vi "TROUBLESHOOTING.vi"() -> ()   [LabVIEW 2017]
uses:
  C:/Users/Admin/Desktop/Sensitive EQE Stuff/S-EQE (YJ)/Mono vi (YJ)/Cornerstone.dll
  Cornerstone.dll
panel:
  out "sendCommand":bool
  out "getResponse":string
  out "Mono Connected?":bool
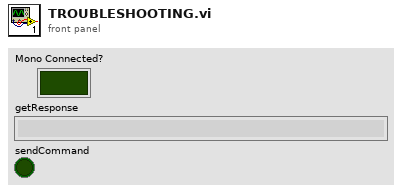
[diagram p1: front panel]
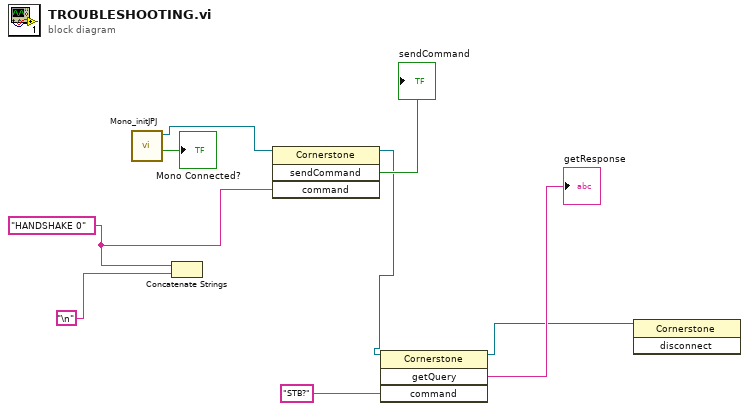
[diagram p0: block diagram]
diagram:
  w1 = "HANDSHAKE 0" ("command")
  n1 = call "Mono_initJPJ.vi"() -> ("Mono Connected?"=→"Mono Connected?":bool, "CmdLib"=w8:refnum<k24>)  [unwired: 9 in, 1 out]
  n2 = Concatenate Strings(w1, "\n") -> ()  [unwired: 1 out]
  n3 = invoke class="Cornerstone" method="sendCommand"(reference=w8, "command"=w1) -> (reference out=w5:refnum<k24>, "sendCommand"=→"sendCommand":bool)  [unwired: 2 in, 2 out]
  n4 = invoke class="Cornerstone" method="getQuery"(reference=w5, "command"="STB?") -> (reference out=w2:refnum<k24>, "getQuery"=→"getResponse":string)  [unwired: 2 in, 2 out]
  n5 = invoke class="Cornerstone" method="disconnect"(reference=w2) -> ()  [unwired: 2 in, 3 out]
